vi "Read Time.vi"(8 "error in (no error)":errorcluster, 11 "ValueChangeMsg in":refnum<class "ValueChangeMsg.lvclass">) -> (0 "error out":errorcluster, 2 "Time":u32, 3 "ValueChangeMsg out":refnum<class "ValueChangeMsg.lvclass">)   [LabVIEW 2018, in "MVA Framework.lvlib" / "ActorEvents.lvlib" / "ValueChangeMsg.lvclass"]
uses:
  ValueChangeMsg.lvclass
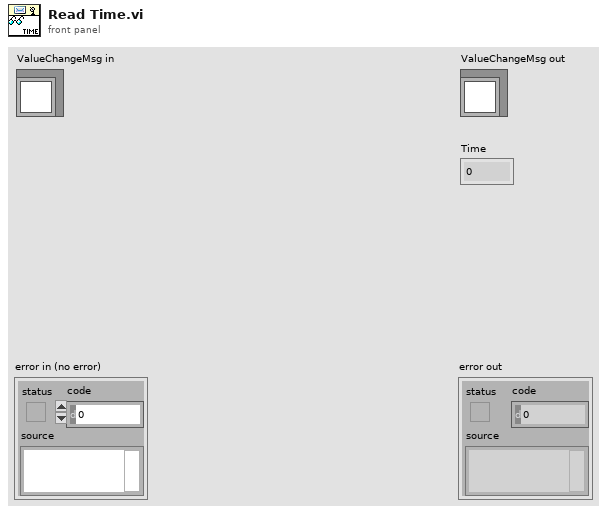
[diagram p1: front panel]
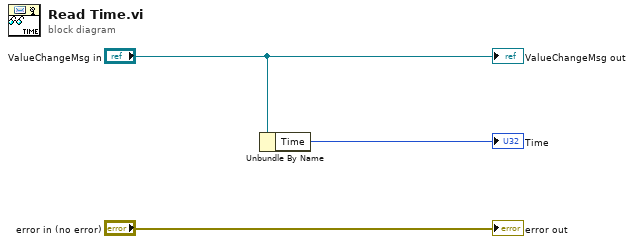
[diagram p0: block diagram]
diagram:
  n1 = Unbundle By Name("ValueChangeMsg in") -> ("Time"=→"Time":u32)
  "error out" <- "error in (no error)"
  "ValueChangeMsg out" <- "ValueChangeMsg in"
